vi "PI_SpeedController.vi"(6 "Current Value (A)":dbl format="%#_13g", 8 "PI Gains":T3 {"dT (s)" format="%#_13g"; "integral gain (s)" format="%#_13g"; "proportional gain (s)" format="%#_13g"}, 9 "Limit Values":T2 {"Upper Limit I Term" format="%#_13g"; "Lower Limit I Term" format="%#_13g"; "Lower Limit Output" format="%#_13g"; "Upper Limit Output" format="%#_13g"}, 10 "Process Variable":dbl, 11 "Setpoint":dbl format="%#_13g") -> (0 "Waveform Chart":T1(graph), 1 "output":dbl, 2 "error":dbl)   [LabVIEW 2015]
uses:
  <vilib>/gmath/NI_Gmath.lvlib
panel:
  in  "Reinitialize?":bool
  out "integrated error":dbl
  out "Feedforward Output":dbl
  in  "Current Axis":dbl[](array[numeric]) format="%_6g"
  in  "Position Axis":dbl[](array[numeric]) format="%_6g"
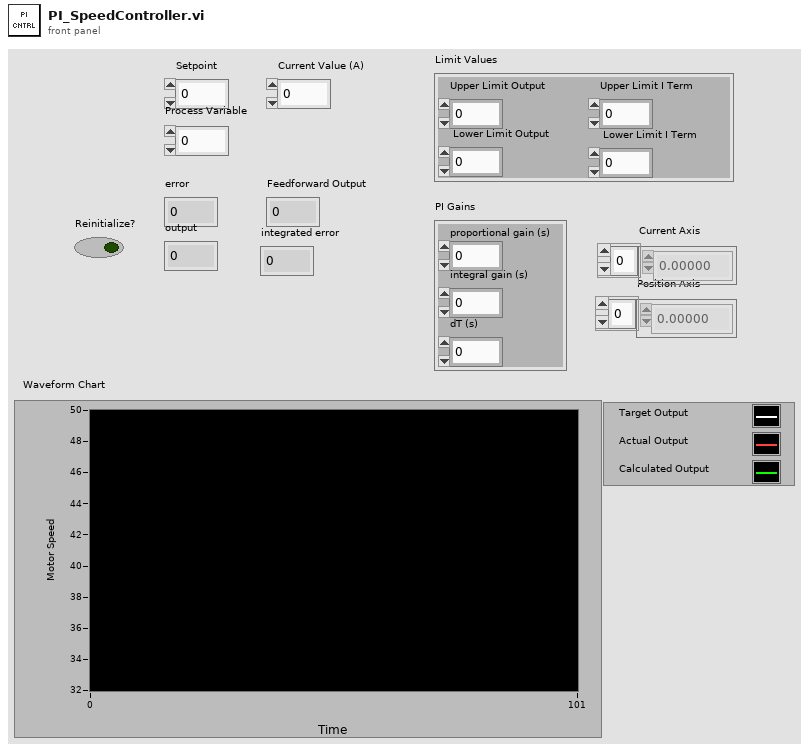
[diagram p1: front panel]
types:
  T1 = cluster{"Setpoint":dbl, "Process Variable":dbl, "Upper Limit Output":dbl}
  T2 = cluster{"Upper Limit Output":dbl, " Lower Limit Output":dbl, " Lower Limit I Term":dbl, "Upper Limit I Term ":dbl}
  T3 = cluster{"proportional gain (s)":dbl, "integral gain (s)":dbl, "dT (s)":dbl}
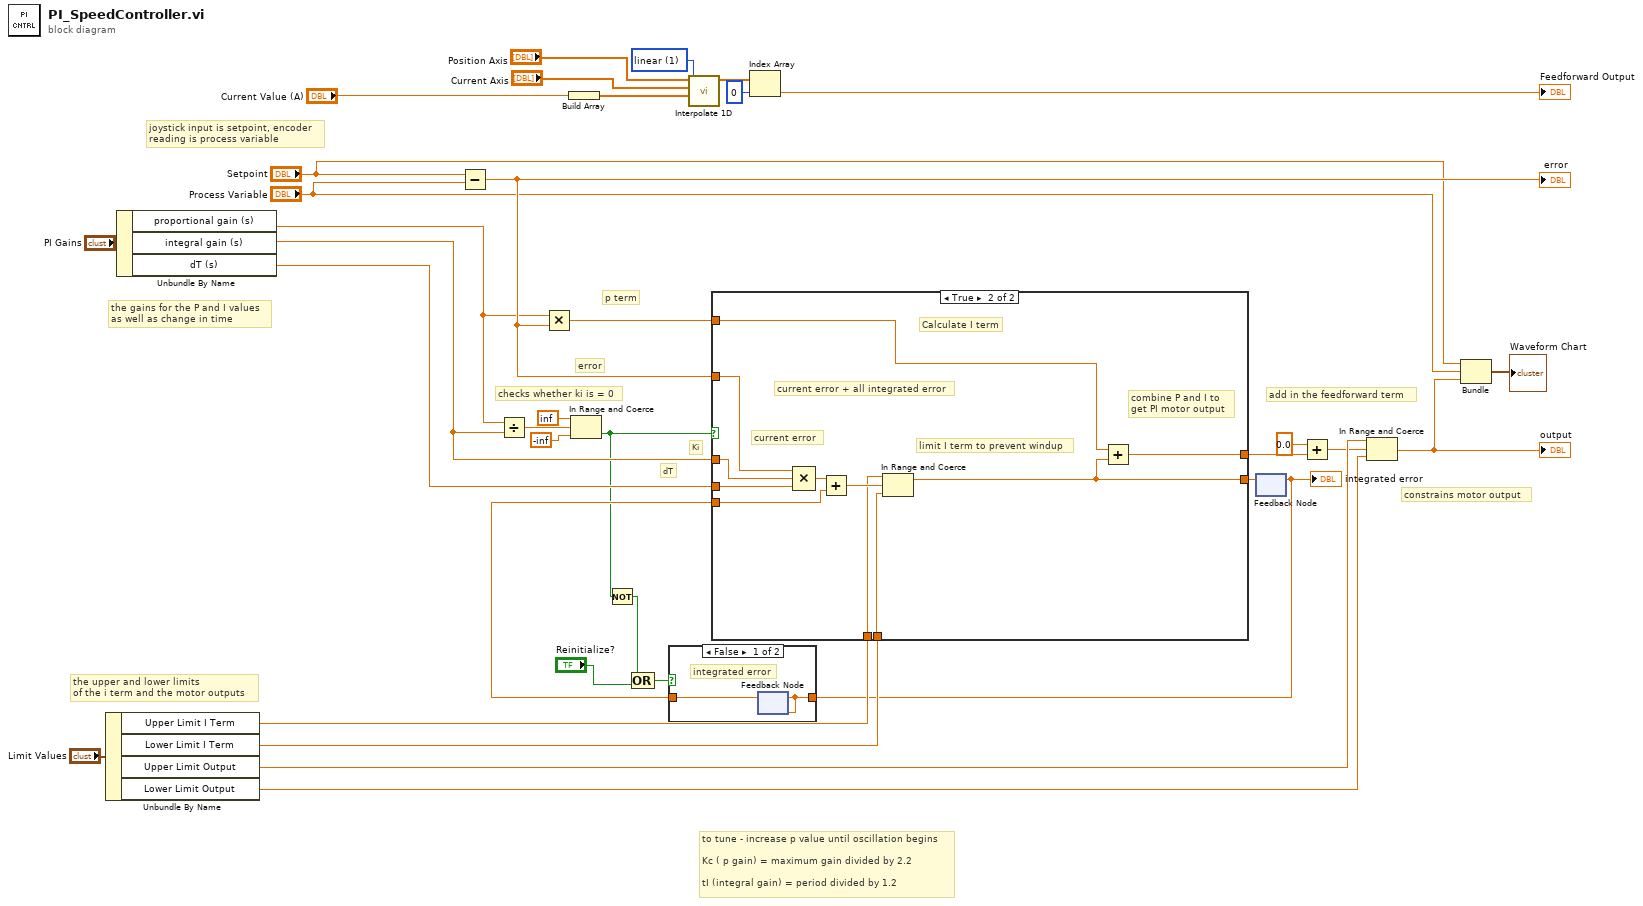
[diagram p0: block diagram]
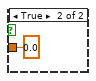
[diagram p2: hidden frame]
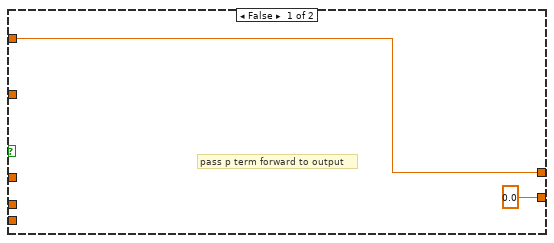
[diagram p3: hidden frame]
diagram:
  w19 = 1 items=["nearest", "linear", "spline", "cubic Hermite", "Lagrange"] ("method")
  # "to tune - increase p value until oscillation begins\n\nKc ( p gain) = maximum gain divided by 2.2\n\ntI (integral gain) = period divided by 1.2"
  # "constrains motor output"
  # "add in the feedforward term"
  # "checks whether ki is = 0"
  # "dT"
  # "Ki"
  # "error"
  # "p term"
  # "the upper and lower limits\nof the i term and the motor outputs"
  # "the gains for the P and I values\nas well as change in time"
  # "joystick input is setpoint, encoder\nreading is process variable"
  n1 = Unbundle By Name("Limit Values") -> ("Upper Limit I Term"=w30:dbl, "Lower Limit I Term"=w29:dbl, "Upper Limit Output"=w27:dbl, "Lower Limit Output"=w26:dbl)
  n2 = Unbundle By Name("PI Gains") -> ("proportional gain (s)"=w34:dbl, "integral gain (s)"=w33:dbl, "dT (s)"=w32:dbl)
  n3 = Subtract(x="Setpoint", y="Process Variable") -> (x-y=w36:dbl)
  "error" <- w36
  n4 = Divide(x=w34, y=w33) -> (x/y=w18:dbl)
  n5 = Multiply(x=w34, y=w36) -> (x*y=w15:dbl)
  n6 = Build Array("Current Value (A)") -> (w20:dbl[])
  n7 = In Range and Coerce(upper limit=inf, x=w18, lower limit=-inf) -> (In Range?=w3:bool)  [unwired: 1 out]
  n8 = Not(x=w3) -> (.not. x?=w2:bool)
  n9 = Compound Arithmetic op=OR(w2, "Reinitialize?") -> (w4:bool)
  n10 = call <vilib>:"Interpolate 1D.vi"("method"=w19, "xi"=w20, "X"="Current Axis", "Y"="Position Axis") -> ("yi"=w23:dbl[])  [unwired: 5 in, 2 out]
  n11 = Index Array(array=w23, index=0) -> (element=→"Feedforward Output":dbl)
  n12 = feedback #1() -> (w5:dbl)  [unwired: 1 in]
  "integrated error" <- w5
  n13 = case shown="False" w4 {
    tunnel: [w38 0.0 ("Upper Limit I Term")] -> w12
    tunnel: w5 -> [w37 _]
    frame False {
      # "integrated error"
      n14 = feedback #2(w37) -> (w38:dbl)
      n15 = feedback-in #2(w37) -> ()
    }
    frame True {
    }
  }
  n16 = case shown="True" w3 {
    tunnel: [w41 w43] -> w13
    tunnel: w15 -> [w41 w46]
    tunnel: w36 -> [_ w52]
    tunnel: w33 -> [_ w51]
    tunnel: w32 -> [_ w50]
    tunnel: [0.0 w42] -> w6
    tunnel: w12 -> [_ w48]
    tunnel: w30 -> [_ w45]
    tunnel: w29 -> [_ w44]
    frame False {
      # "pass p term forward to output"
    }
    frame True {
      # "limit I term to prevent windup"
      # "combine P and I to \nget PI motor output"
      # "current error"
      # "current error + all integrated error"
      # "Calculate I term"
      n17 = Compound Arithmetic op=MULTIPLY(w52, w51, w50) -> (w49:dbl)
      n18 = Add(x=w49, y=w48) -> (x+y=w47:dbl)
      n19 = In Range and Coerce(upper limit=w45, x=w47, lower limit=w44) -> (coerced(x)=w42:dbl)  [unwired: 1 out]
      n20 = Add(x=w46, y=w42) -> (x+y=w43:dbl)
    }
  }
  n21 = feedback-in #1(w6) -> ()
  n22 = Add(x=0.0, y=w13) -> (x+y=w14:dbl)
  n23 = In Range and Coerce(upper limit=w27, x=w14, lower limit=w26) -> (coerced(x)=w8:dbl)  [unwired: 1 out]
  "output" <- w8
  n24 = Bundle("Setpoint"="Setpoint", "Process Variable"="Process Variable", "Upper Limit Output"=w8) -> (→"Waveform Chart":T1)  [unwired: 1 in]
